vi "Accounts_FGV.vi"(9 "User Input":string, 11 "Access mode":T1) -> (2 "Find":bool, 3 "User Info":string[](array[string]))   [LabVIEW 2015]
uses:
  Controls/AccessModeFGV.ctl
  <vilib>/Utility/file.llb/Read Delimited Spreadsheet (string).vi
panel:
  out "all rows":string[][](array[string])
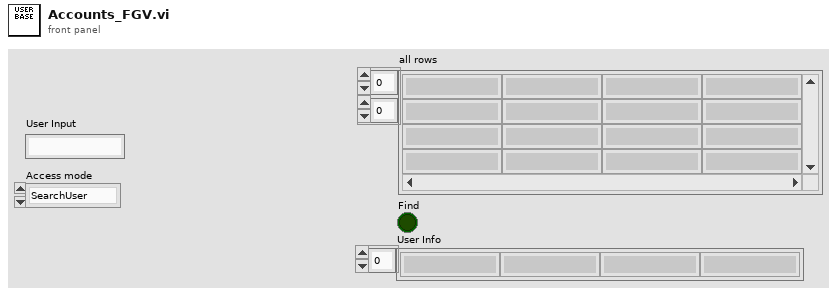
[diagram p1: front panel]
types:
  T1 = typedef "AccessModeFGV.ctl" = enum16{"SearchUser", "Deposite", "Withdraw", "Fast Cash $50", "Balance Inquiry"}
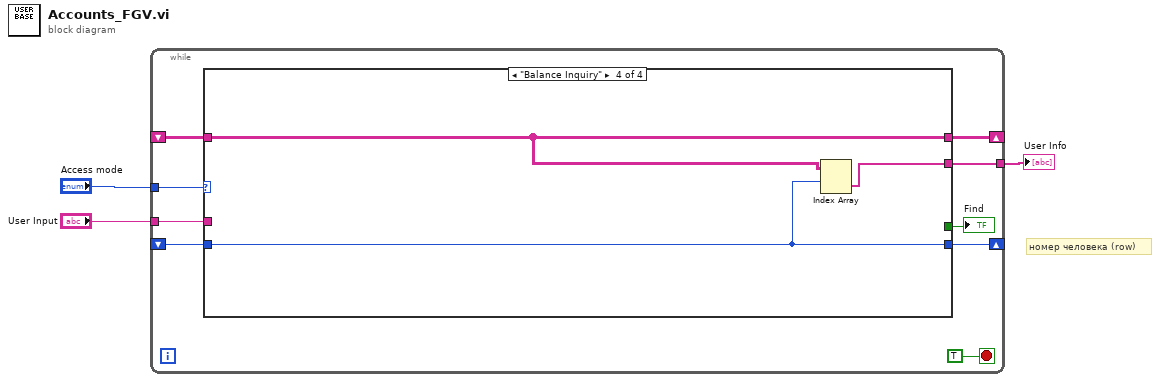
[diagram p0: block diagram]
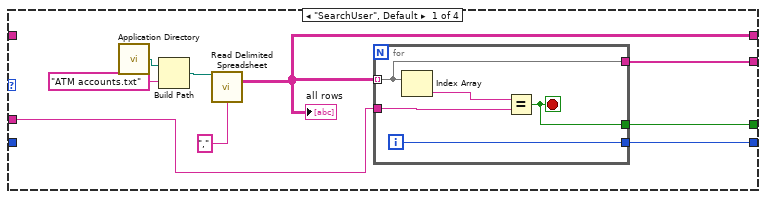
[diagram p2: hidden frame]
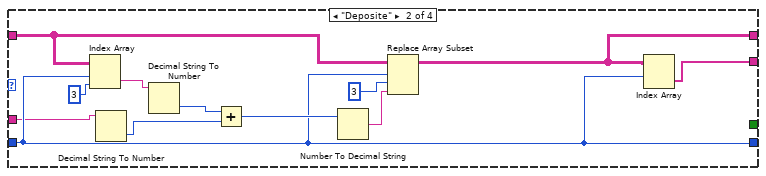
[diagram p3: hidden frame]
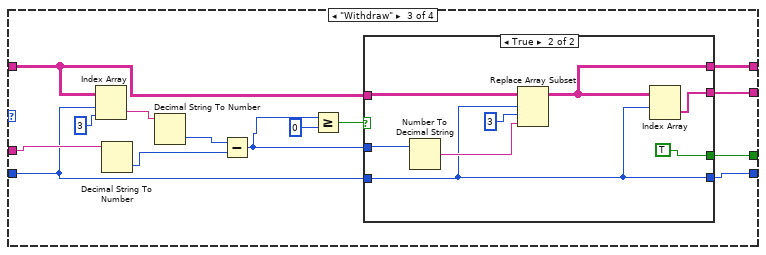
[diagram p4: hidden frame]
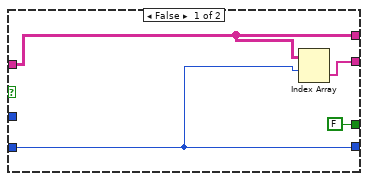
[diagram p5: hidden frame]
diagram:
  # "номер человека (row)"
  n1 = while {
    shift-right: [w8] -> _
    shift-left: _ -> [w10]
    tunnel: "Access mode" -> [w12]
    tunnel: [w9] -> w2
    shift-right: [w7] -> _
    shift-left: _ -> [w6]
    tunnel: "User Input" -> [w5]
    stop <- TRUE stop-if-true
    n2 = case shown="\"Balance Inquiry\"" w12 {
      tunnel: [w18 w30 w47 w66] -> w9
      tunnel: w10 -> [_ w35 w45 w67]
      tunnel: [w16 w31 w46 w67] -> w8
      tunnel: [w15 w29 w39 w65] -> w7
      tunnel: w6 -> [_ w29 w40 w65]
      tunnel: w5 -> [w14 w28 w48 _]
      tunnel: [w13 _ w41 _] -> w4
      frame "SearchUser", Default {
        n3 = call <vilib>:"Application Directory.vi"() -> ("Application Directory"=w17:path)
        n4 = Build Path(base path=w17, name or relative path="ATM accounts.txt") -> (appended path=w20:path)
        n5 = call-poly <vilib>:"Read Delimited Spreadsheet.vi"("file path (dialog if empty)"=w20, "delimiter (\\t)"="," ("delimiter (\\t)")) -> ("all rows"=w16:string[][])  [unwired: 8 in, 5 out]
        "all rows" <- w16
        n6 = for {
          tunnel: w16 -> [w25] mode=indexing
          tunnel: [w26] -> w15
          tunnel: [w25] -> w18
          tunnel: [w24] -> w13
          tunnel: w14 -> [w22]
          i -> [w26]
          stop <- w24 stop-if-true
          n7 = Index Array(array=w25) -> (element=w23:string)  [unwired: 1 in]
          n8 = Equal?(x=w23, y=w22) -> (x = y?=w24:bool)
        }
      }
      frame "Deposite" {
        n9 = Index Array(array=w35, index (row)=w29, index (col)=3 ("index")) -> (element=w38:string)
        n10 = Decimal String To Number(string=w28) -> (number=w27:i32)  [unwired: 2 in, 1 out]
        n11 = Decimal String To Number(string=w38) -> (number=w37:i32)  [unwired: 2 in, 1 out]
        n12 = Add(x=w37, y=w27) -> (x+y=w32:i32)
        n13 = Number To Decimal String(number=w32) -> (decimal integer string=w33:string)  [unwired: 1 in]
        n14 = Replace Array Subset(array=w35, new element=w33, index (row)=w29, index (col)=3 ("disabled index (col)")) -> (w31:string[][])
        n15 = Index Array(array=w31, index (row)=w29) -> (element=w30:string[])  [unwired: 1 in]
      }
      frame "Withdraw" {
        n16 = Index Array(array=w45, index (row)=w40, index (col)=3 ("index")) -> (element=w52:string)
        n17 = Decimal String To Number(string=w48) -> (number=w49:i32)  [unwired: 2 in, 1 out]
        n18 = Decimal String To Number(string=w52) -> (number=w51:i32)  [unwired: 2 in, 1 out]
        n19 = Subtract(x=w51, y=w49) -> (x-y=w43:i32)
        n20 = Greater Or Equal?(x=w43, y=0) -> (x >= y?=w44:bool)
        n21 = case shown="True" w44 {
          tunnel: w43 -> [_ w64]
          tunnel: [w55 w61] -> w47
          tunnel: [w56 w60] -> w46
          tunnel: w45 -> [w56 w59]
          tunnel: w40 -> [w54 w57]
          tunnel: [FALSE TRUE] -> w41
          tunnel: [w54 w57] -> w39
          frame False {
            n22 = Index Array(array=w56, index (row)=w54) -> (element=w55:string[])  [unwired: 1 in]
          }
          frame True {
            n23 = Number To Decimal String(number=w64) -> (decimal integer string=w63:string)  [unwired: 1 in]
            n24 = Replace Array Subset(array=w59, new element=w63, index (row)=w57, index (col)=3 ("disabled index (col)")) -> (w60:string[][])
            n25 = Index Array(array=w60, index (row)=w57) -> (element=w61:string[])  [unwired: 1 in]
          }
        }
      }
      frame "Balance Inquiry" {
        n26 = Index Array(array=w67, index (row)=w65) -> (element=w66:string[])  [unwired: 1 in]
      }
    }
    "Find" <- w4
  }
  "User Info" <- w2
